vi "Utility - Process ROIs.vi"(8 "error in (no error)":errorcluster, 9 "Overlay?":bool, 10 "QSM_ShiftRegister_TEST in":T2 {"ROI Process"."Particle Variables" items=["Center of Mass X", "Center of Mass Y", "First Pixel X", "First Pixel Y", "Bounding Rect Left", "Bounding Rect Top", "Bounding Rect Right", "Bounding Rect Bottom", "Max Feret Diameter Start X", "Max Feret Diameter Start Y", "Max Feret Diameter End X", "Max Feret Diameter End Y", "Max Horiz. Segment Length Left", "Max Horiz. Segment Length Right", "Max Horiz. Segment Length Row", "-", "Bounding Rect Width", "Bounding Rect Height", "Bounding Rect Diagonal", "Perimeter", "Convex Hull Perimeter", "Holes' Perimeter", "Max Feret Diameter", "Equivalent Ellipse Major Axis", "Equivalent Ellipse Minor Axis", "Equivalent Ellipse Minor Axis (Feret)", "Equivalent Rect Long Side", "Equivalent Rect Short Side", "Equivalent Rect Diagonal", "Equivalent Rect Short Side (Feret)", "Average Horiz. Segment Length", "Average Vert. Segment Length", "Hydraulic Radius", "Waddel Disk Diameter", "-", "Area", "Holes' Area", "Particle & Holes' Area", "Convex Hull Area", "Image Area", "-", "Number of Holes", "Number of Horiz. Segments", "Number of Vert. Segments", "-", "Orientation", "Max Feret Diameter Orientation", "-", "% Area/Image Area", "% Area/(Particle & Holes' Area)", "Ratio of Equivalent Ellipse Axes", "Ratio of Equivalent Rect Sides", "-", "Elongation Factor", "Compactness Factor", "Heywood Circularity Factor", "Type Factor", "-", "Sum X", "Sum Y", "Sum XX", "Sum XY", "Sum YY", "Sum XXX", "Sum XXY", "Sum XYY", "Sum YYY", "-", "Moment of Inertia XX", "Moment of Inertia XY", "Moment of Inertia YY", "Moment of Inertia XXX", "Moment of Inertia XXY", "Moment of Inertia XYY", "Moment of Inertia YYY", "Norm. Moment of Inertia XX", "Norm. Moment of Inertia XY", "Norm. Moment of Inertia YY", "Norm. Moment of Inertia XXX", "Norm. Moment of Inertia XXY", "Norm. Moment of Inertia XYY", "Norm. Moment of Inertia YYY", "Hu Moment 1", "Hu Moment 2", "Hu Moment 3", "Hu Moment 4", "Hu Moment 5", "Hu Moment 6", "Hu Moment 7"]; "ROI Process"."Particle Measurements (Pixels)" format="%.2f"; "ROI Process"."ROIS"."Contours"."Type" items=["No Selection", "Point", "Line", "Rectangle", "Oval", "Polygon", "Freehand Region", "Annulus", "Unused2", "Unused3", "Broken Line", "Freehand Line", "Rotated Rectangle"]; "Single Image Results"."ROI Results"."LIMLOCALMETADATA"."dTimeMSec" format="%.2f"}, 11 "Original Image In":T1) -> (0 "error out":errorcluster, 1 "ROI Calculation":dbl[](array[numeric]), 2 "ROI Snippet Out":T1, 3 "Original Image with overlays out":T1)   [LabVIEW 2014, in "TestQSM.lvlib"]
uses:
  TestQSM.lvlib
  Controls/QSM_ShiftRegister.ctl
  QueueMaintenance/TypeDef/QSMRef_ALL.ctl
  Queue_TESTGUIUPDATE/Controls/QSM_Reference.ctl
  Queue_TESTGUIUPDATE/Controls/QSM_DataType.ctl
  Queue_TESTGUIUPDATE/Controls/QSM_RunStates.ctl
  Controls/QSM_Reference.ctl
  Controls/QSM_DataType.ctl
  Controls/QSM_RunStates.ctl
  Custom Controls/cluster - Image Results.ctl
  ND2_Reader_32bit/controls/cluster_LIMLOCALMETADATA.ctl
  <vilib>/vision/Image Controls.llb/IMAQ Image.ctl
  Queue_TESTGUIUPDATE/GUIUpdateQSM.lvlib
  QueueMaintenance/QueueMaintenance.lvlib
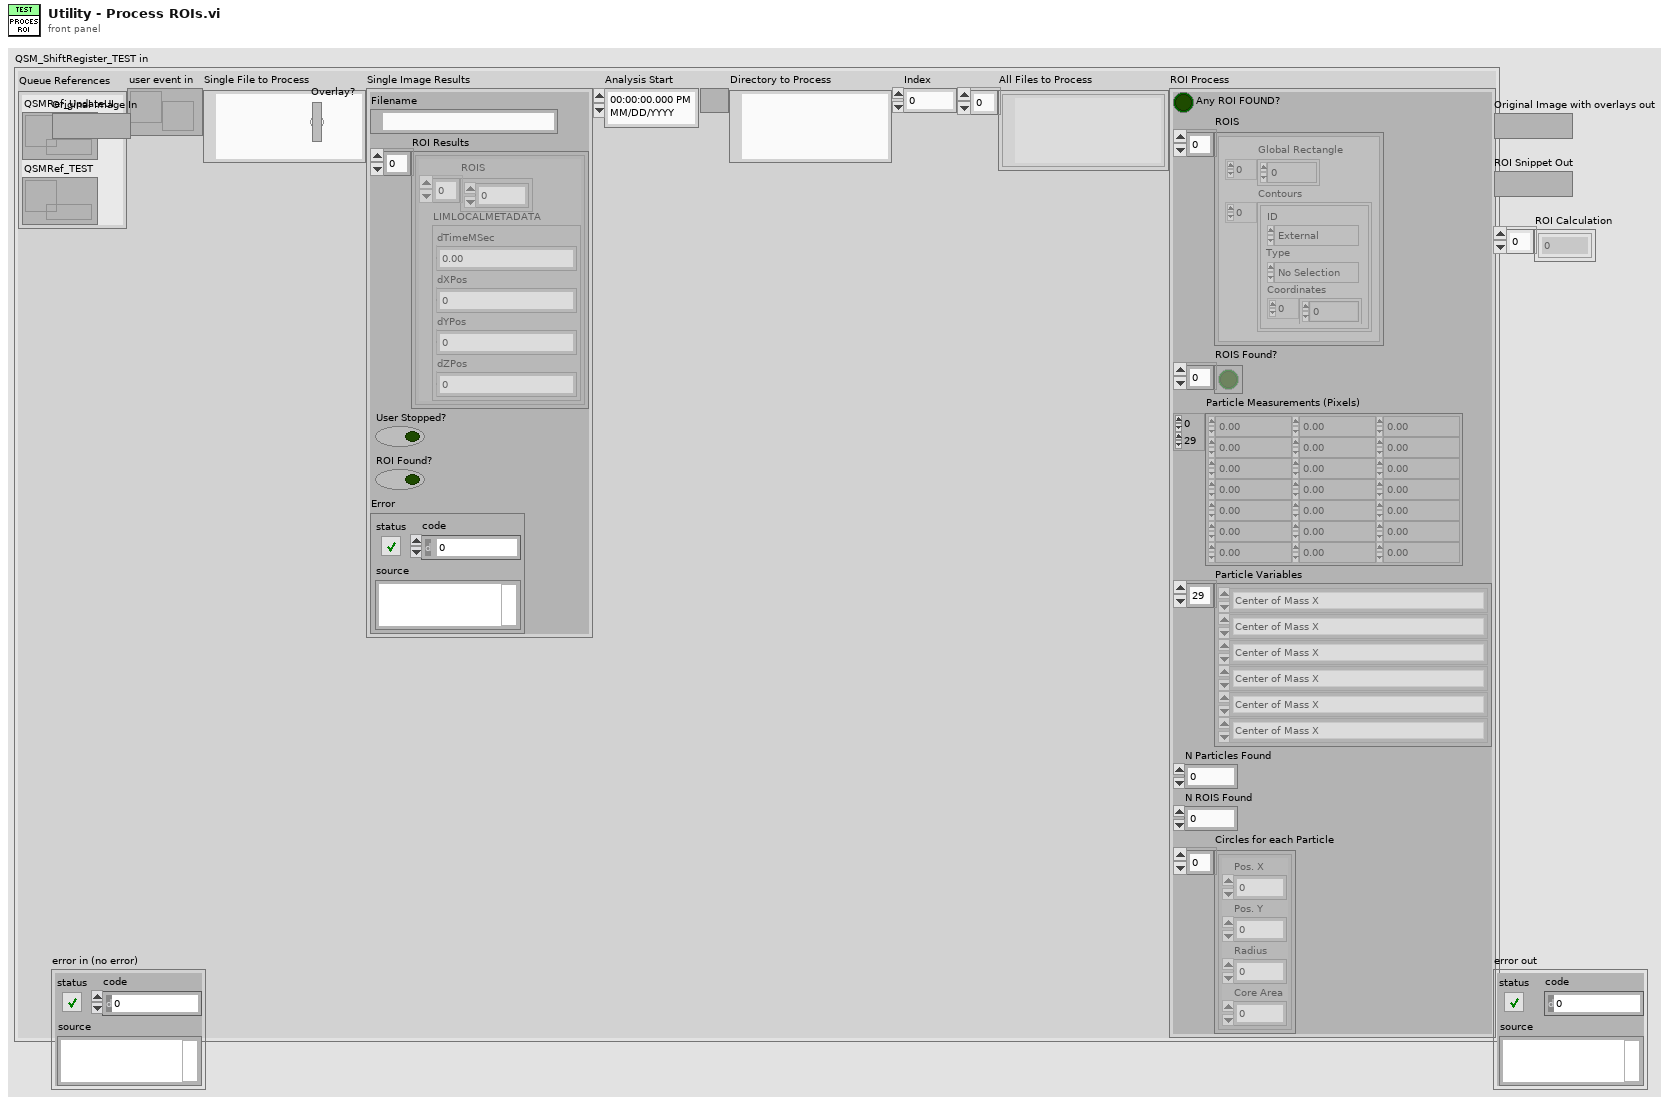
[diagram p1: front panel]
types:
  T1 = typedef "IMAQ Image.ctl" = refnum<image>
  T2 = typedef "TestQSM.lvlib/QSM_ShiftRegister.ctl" = cluster{"Queue References":T3, "user event in":refnum<user-event>, "Single File to Process":path, "Single Image Results":T6, "Analysis Start":timestamp, "Directory to Process":path, "Index":i32, "All Files to Process":path[], "ROI Process":cluster{"Any ROI FOUND?":bool, "ROIS":T8[], "ROIS Found?":bool[], "Particle Measurements (Pixels)":dbl[][], "Particle Variables":i32[], "N Particles Found":i32, "N ROIS Found":i32, "Circles for each Particle":cluster{"Pos. X":i32, "Pos. Y":i32, "Radius":i32, "Core Area":i32}[]}}
  T3 = typedef "QueueMaintenance.lvlib/QSMRef_ALL.ctl" = cluster{"QSMRef_UpdateUI":T4, "QSMRef_TEST":T5}
  T4 = typedef "GUIUpdateQSM.lvlib/QSM_Reference.ctl" = refnum<queue>
  T5 = typedef "TestQSM.lvlib/QSM_Reference.ctl" = refnum<queue>
  T6 = typedef "cluster - Image Results.ctl" = cluster{"Filename":path, "ROI Results":cluster{"ROIS":dbl[], "LIMLOCALMETADATA":T7}[], "User Stopped?":bool, "ROI Found?":bool, "Error":errorcluster}
  T7 = typedef "cluster_LIMLOCALMETADATA.ctl" = cluster{"dTimeMSec":dbl, "dXPos":dbl, "dYPos":dbl, "dZPos":dbl}
  T8 = typedef "ROI Descriptor" = cluster{"Global Rectangle":i32[], "Contours":cluster{"ID":enum32{"External", "Internal"}, "Type":u32, "Coordinates":i32[]}[]}
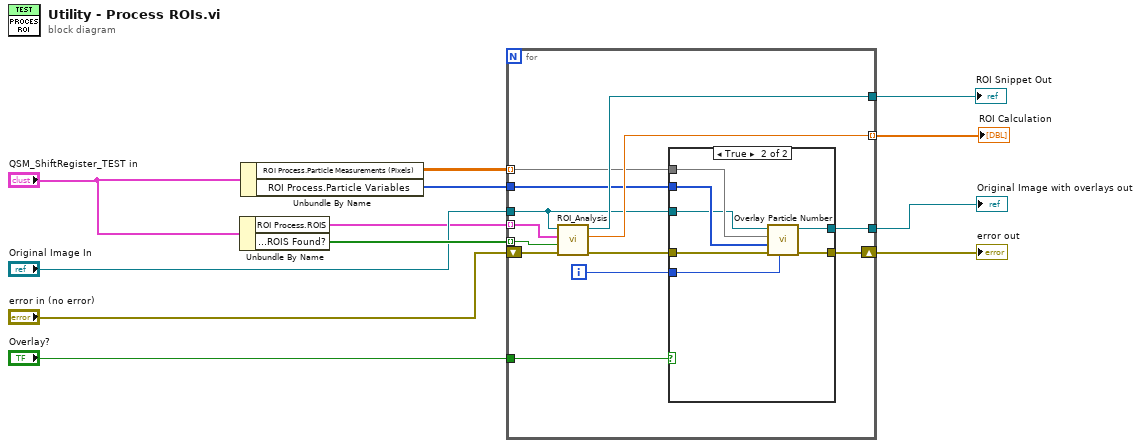
[diagram p0: block diagram]
diagram:
  n1 = Unbundle By Name("QSM_ShiftRegister_TEST in") -> ("ROI Process.ROIS"=w5:T8[], "ROI Process.ROIS Found?"=w12:bool[])
  n2 = Unbundle By Name("QSM_ShiftRegister_TEST in") -> ("ROI Process.Particle Measurements (Pixels)"=w3:dbl[][], "ROI Process.Particle Variables"=w2:i32[])
  n3 = for {
    tunnel: w5 -> [w25] mode=indexing
    tunnel: "Original Image In" -> [w16]
    tunnel: [w23] -> w9
    tunnel: [w22] -> w8 mode=indexing
    shift-right: [w14] -> w6
    shift-left: "error in (no error)" -> [w24]
    tunnel: w12 -> [w21] mode=indexing
    tunnel: [w20] -> w11
    tunnel: w3 -> [w18] mode=indexing
    tunnel: w2 -> [w17]
    tunnel: "Overlay?" -> [w13]
    i -> [w19]
    n4 = call "ROI_Analysis.vi"("error in (no error)"=w24, "Valid ROI"=w21, "ROI"=w25, "Image In"=w16) -> ("error out"=w15:errorcluster, "ROI Results"=w22:dbl, "ROI Snippet Out"=w23:T1)  [unwired: 5 in]
    n5 = case shown="True" w13 {
      tunnel: [w27 w34] -> w20
      tunnel: w19 -> [_ w33]
      tunnel: w18 -> [_ w32]
      tunnel: w17 -> [_ w31]
      tunnel: w16 -> [w27 w30]
      tunnel: w15 -> [w26 w29]
      tunnel: [w26 w28] -> w14
      frame False {
      }
      frame True {
        n6 = call "Overlay Particle Number.vi"("Particle Index"=w33, "error in"=w29, "Particle Variables"=w31, "Particle Measurements (Pixels)"=w32, "Image"=w30) -> ("error out"=w28:errorcluster, "Image Out"=w34:T1)  [unwired: 5 in]
      }
    }
  }
  "Original Image with overlays out" <- w11
  "ROI Snippet Out" <- w9
  "ROI Calculation" <- w8
  "error out" <- w6
